vi "Create.vi"(8 "error in (no error)":errorcluster, 9 "Row":i32, 10 "Col Offset":i32, 11 "String":string) -> (0 "error out":errorcluster, 2 "Offset Past Number":i32, 3 "Number":refnum<class "Number.lvclass">)   [LabVIEW 2020, in "Number.lvclass"]
uses:
  Number.lvclass
  Number.lvclass/Number.ctl
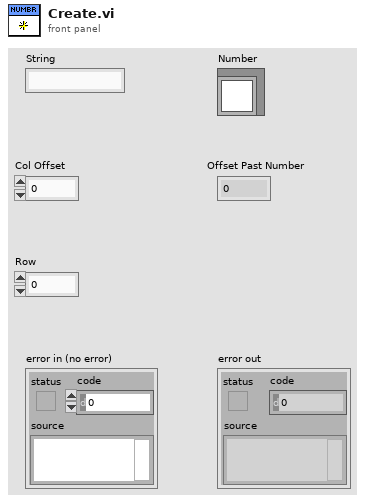
[diagram p1: front panel]
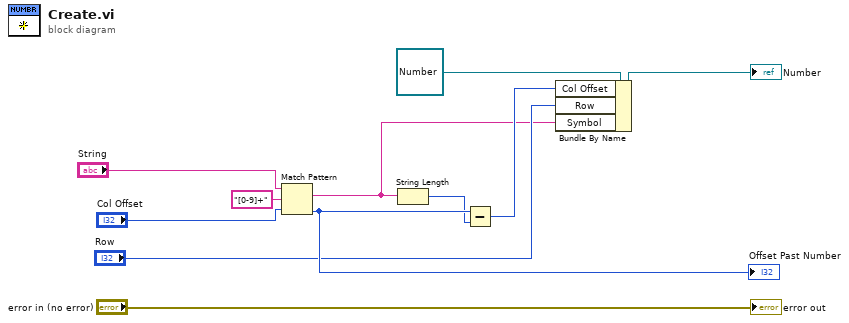
[diagram p0: block diagram]
diagram:
  n1 = Match Pattern(string="String", regular expression="[0-9]+", offset (0)="Col Offset") -> (match substring=w1:string, offset past match=w5:i32)  [unwired: 2 out]
  "Offset Past Number" <- w5
  n2 = String Length(string=w1) -> (length=w4:i32)
  n3 = Subtract(x=w5, y=w4) -> (x-y=w3:i32)
  n4 = Bundle By Name(cluster=refnum<class "Number.lvclass"> refnum ("Number"), "Col Offset"=w3, "Row"="Row", "Symbol"=w1) -> (→"Number":refnum<class "Number.lvclass">)
  "error out" <- "error in (no error)"
